vi "test15-LosslessRegisterStatusMultipleTimes.vi"(8 "error in (no error)":errorcluster, 11 "TestCase in":refnum<class "testcase-CSMBroadcast.lvclass">) -> (0 "error out":errorcluster, 3 "TestCase out":refnum<class "testcase-CSMBroadcast.lvclass">)   [LabVIEW 2017, in "testcase-CSMBroadcast.lvclass"]
uses:
  testcase-CSMBroadcast.lvclass
  bc269a46-fbd8-4fbd-ac76-06990d02385a.vi
  8d37a2f4-20d8-4102-818c-5a8acec6f80e.vi
  src/user.lib/_NEVSTOP/Communicable State Machine(CSM)/AdvanceAPI/CSM - Get Module Attribute.vi
  <vilib>/addons/_JKI Toolkits/VI Tester/TestCase.llb/TestCase.lvclass
  src/user.lib/_NEVSTOP/Communicable State Machine(CSM)/Communicable State Machine.lvlib
  CSM/CSM-Testcase.lvlib
  C:/Program Files (x86)/National Instruments/LabVIEW 2017/vi.lib/addons/_JKI Toolkits/VI Tester/TestCase.llb/TestCase.lvclass
panel:
  out "LoopCount":i32
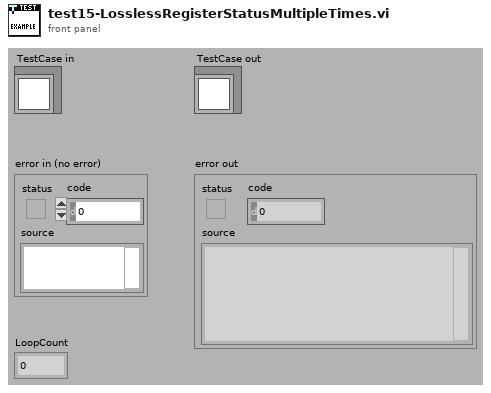
[diagram p1: front panel]
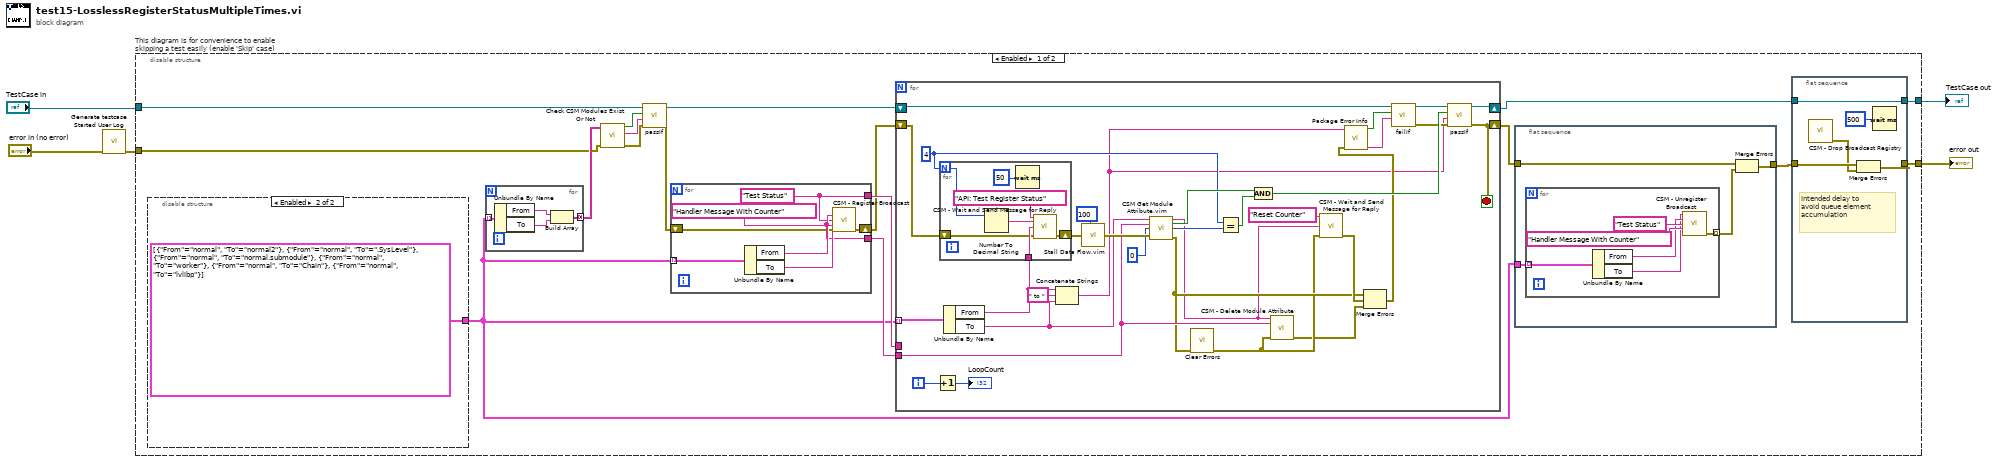
[diagram p0: block diagram]
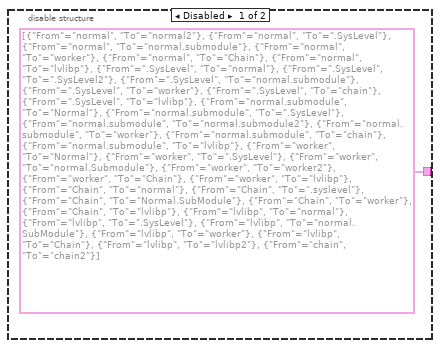
[diagram p2: hidden frame]
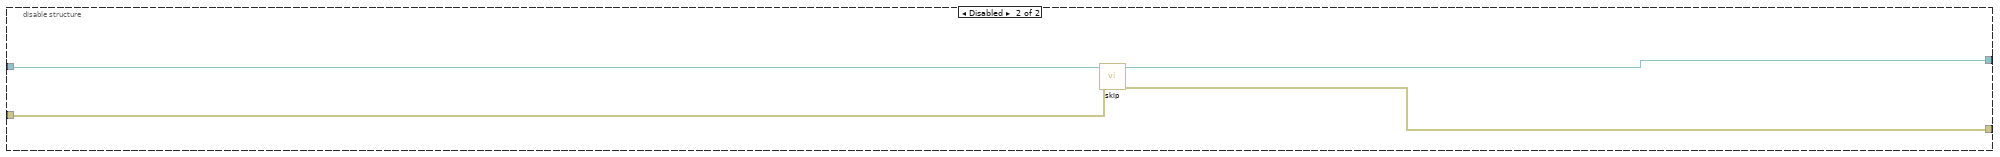
[diagram p3: hidden frame]
diagram:
  n1 = call "Generate testcase Started User Log.vi"("Error In"="error in (no error)") -> ("error out"=w1:errorcluster)  [unwired: 10 in]
  n2 = disable-structure "This diagram is for convenience to enable skipping a test easily (enable 'Skip' case)" shown="Enabled" {
    disable-tunnel: "TestCase in" -> [w11 w93]
    disable-tunnel: [w17 w91] -> w3
    disable-tunnel: [w20 w92] -> w2
    disable-tunnel: w1 -> [w9 w90]
    frame Enabled {
      n3 = disable-structure shown="Enabled" {
        disable-tunnel: [cluster{"From":string, "To":string}[] [{"From"="normal", "To"="normal2"}, {"From"="normal", "To"=".SysLevel"}, {"From"="normal", "To"="normal.submodule"}, {"From"="normal", "To"="worker"}, {"From"="normal", "To"="Chain"}, {"From"="normal", "To"="lvlibp"}, {"From"=".SysLevel", "To"="normal"}, {"From"=".SysLevel", "To"=".SysLevel2"}, {"From"=".SysLevel", "To"="normal.submodule"}, {"From"=".SysLevel", "To"="worker"}, {"From"=".SysLevel", "To"="chain"}, {"From"=".SysLevel", "To"="lvlibp"}, {"From"="normal.submodule", "To"="Normal"}, {"From"="normal.submodule", "To"=".SysLevel"}, {"From"="normal.submodule", "To"="normal.submodule2"}, {"From"="normal.submodule", "To"="worker"}, {"From"="normal.submodule", "To"="chain"}, {"From"="normal.submodule", "To"="lvlibp"}, {"From"="worker", "To"="Normal"}, {"From"="worker", "To"=".SysLevel"}, {"From"="worker", "To"="normal.Submodule"}, {"From"="worker", "To"="worker2"}, {"From"="worker", "To"="Chain"}, {"From"="worker", "To"="lvlibp"}, {"From"="Chain", "To"="normal"}, {"From"="Chain", "To"=".syslevel"}, {"From"="Chain", "To"="Normal.SubModule"}, {"From"="Chain", "To"="worker"}, {"From"="Chain", "To"="lvlibp"}, {"From"="lvlibp", "To"="normal"}, {"From"="lvlibp", "To"=".SysLevel"}, {"From"="lvlibp", "To"="normal.SubModule"}, {"From"="lvlibp", "To"="worker"}, {"From"="lvlibp", "To"="Chain"}, {"From"="lvlibp", "To"="lvlibp2"}, {"From"="chain", "To"="chain2"}] cluster{"From":string, "To":string}[] [{"From"="normal", "To"="normal2"}, {"From"="normal", "To"=".SysLevel"}, {"From"="normal", "To"="normal.submodule"}, {"From"="normal", "To"="worker"}, {"From"="normal", "To"="Chain"}, {"From"="normal", "To"="lvlibp"}]] -> w6
        frame Disabled {
        }
        frame Enabled {
        }
      }
      n4 = for {
        tunnel: w6 -> [w28] mode=indexing
        tunnel: [w25] -> w14 mode=concatenating
        n5 = Unbundle By Name(w28) -> ("From"=w27:string, "To"=w26:string)
        n6 = Build Array(w27, w26) -> (w25:string[])
      }
      n7 = call "Check CSM Modules Exist Or Not.vi"("error in"=w9, "CSM names in"=w14) -> ("error out"=w12:errorcluster, "Debug string"=w13:string, "All Modules Exist?"=w15:bool)  [unwired: 7 in]
      n8 = call-dynamic "passIf.vi"("error in (no error)"=w12, "message (\"\")"=w13, "pass"=w15, "TestCase in"=w11) -> ("error out"=w8:errorcluster, "TestCase out"=w10:refnum<class "testcase-CSMBroadcast.lvclass">)  [unwired: 6 in]
      n9 = for {
        tunnel: w6 -> [w45] mode=indexing
        tunnel: [w41] -> w19
        tunnel: [w40] -> w16
        shift-right: [w42] -> w7
        shift-left: w8 -> [w39]
        w40 = "Handler Message With Counter" ("Response Message (If \"\", Same as Source Message)")
        w41 = "Test Status" ("Status")
        n10 = Unbundle By Name(w45) -> ("From"=w44:string, "To"=w43:string)
        n11 = call "CSM - Register Broadcast.vi"("CSM Name(Empty for Broadcast Event)"=w43, "Source CSM Name (* as Default)"=w44, "Trigger"=w41, "API (If \"\", Same as Trigger)"=w40, "Error In"=w39) -> ("error out"=w42:errorcluster)  [unwired: 9 in, 1 out]
      }
      n12 = for {
        tunnel: w6 -> [w82] mode=indexing
        shift-right: [w77] -> w18
        shift-left: w10 -> [w60]
        shift-right: [w75] -> w22
        shift-left: w7 -> [w63]
        tunnel: w19 -> [_]
        tunnel: w16 -> [w74]
        i -> [w73]
        stop <- w75 stop-if-true
        w69 = 4
        n13 = Increment(x=w73) -> (x+1=→"LoopCount":i32)
        n14 = Unbundle By Name(w82) -> ("From"=w56:string, "To"=w55:string)
        n15 = for {
          N: w69 -> [w84]
          tunnel: w56 -> [w87]
          shift-right: [w88] -> w81
          shift-left: w63 -> [w86]
          n16 = Number To Decimal String(number=w84) -> (decimal integer string=w85:string)  [unwired: 1 in]
          n17 = Wait (ms)(milliseconds to wait=u32 50) -> ()  [unwired: 1 out]
          n18 = call "CSM - Wait and Send Message for Reply.vi"("State"="API: Test Register Status", "Arguments (\"\")"=w85, "Target Module"=w87, "Error In (No Error)"=w86) -> ("error out"=w88:errorcluster)  [unwired: 8 in, 3 out]
        }
        n19 = Concatenate Strings(w56, " to " ("string"), w55) -> (w53:string)
        n20 = call "Stall Data Flow.vim"("value in"=w81, "milliseconds to wait"=u32 100) -> ("value out"=w79:errorcluster)  [unwired: 1 out]
        n21 = call "CSM Get Module Attribute.vim"("CSM Name"=w55, "Attribute"=w74, "Default Value (Empty Variant)"=u32 0, "Error In"=w79) -> ("CSM Name (Dup)"=w51:string, "Found"=w78:bool, "Value"=w70:u32, "error out"=w66:errorcluster)  [unwired: 7 in, 1 out]
        n22 = call <vilib>:"Clear Errors.vi"("error in (no error)"=w66) -> ("error out"=w65:errorcluster)  [unwired: 5 in, 1 out]
        n23 = Equal?(x=w69, y=w70) -> (x = y?=w68:bool)
        n24 = Compound Arithmetic op=AND(w78, w68) -> (w76:bool)
        n25 = call "CSM - Delete Module Attribute.vi"("CSM Name"=w51, "Attribute"=w74, "Error In"=w65) -> ("error out"=w64:errorcluster)  [unwired: 9 in, 3 out]
        n26 = call "CSM - Wait and Send Message for Reply.vi"("State"="Reset Counter", "Target Module"=w51, "Error In (No Error)"=w65) -> ("error out"=w67:errorcluster)  [unwired: 9 in, 3 out]
        n27 = Merge Errors(w66, w67, w64) -> (w57:errorcluster)
        n28 = call "Package Error Info.vi"("error in"=w57, "String in"=w53) -> ("packed error info out"=w61:string, "error status"=w62:bool)  [unwired: 8 in]
        n29 = call-dynamic "failIf.vi"("message (\"\")"=w61, "fail"=w62, "TestCase in"=w60) -> ("error out"=w58:errorcluster, "TestCase out"=w59:refnum<class "testcase-CSMBroadcast.lvclass">)  [unwired: 7 in]
        n30 = call-dynamic "passIf.vi"("error in (no error)"=w58, "message (\"\")"=w53, "pass"=w76, "TestCase in"=w59) -> ("error out"=w75:errorcluster, "TestCase out"=w77:refnum<class "testcase-CSMBroadcast.lvclass">)  [unwired: 6 in]
      }
      n31 = flat-sequence {
        tunnel: w6 -> [w29]
        tunnel: w22 -> [w32]
        tunnel: [w31] -> w21
        frame #0 {
          n32 = for {
            tunnel: w29 -> [w33] mode=indexing
            tunnel: [w34] -> w30 mode=indexing
            n33 = Unbundle By Name(w33) -> ("From"=w36:string, "To"=w35:string)
            n34 = call "CSM - Unregister Broadcast.vi"("CSM Name(Empty for Broadcast Event)"=w35, "Source CSM Name (* as Default)"=w36, "Trigger"="Test Status" ("Status"), "API (\"*\" as Default)"="Handler Message With Counter" ("Response Message (If \"\", Same as Source Message)")) -> ("error out"=w34:errorcluster)  [unwired: 10 in, 1 out]
          }
          n35 = Merge Errors(w32, w30) -> (w31:errorcluster)
        }
      }
      n36 = flat-sequence {
        tunnel: w21 -> [w50]
        tunnel: [w49] -> w20
        tunnel: [w48] -> w17
        tunnel: w18 -> [w48]
        frame #0 {
          # "Intended delay to \navoid queue element\naccumulation"
          n37 = call "CSM - Drop Broadcast Registry.vi"() -> ("error out"=w47:errorcluster)  [unwired: 15 in]
          n38 = Merge Errors(w50, w47) -> (w49:errorcluster)
          n39 = Wait (ms)(milliseconds to wait=u32 500) -> ()  [unwired: 1 out]
        }
      }
    }
    frame Disabled {
      # "skip test result while test is under development"
      n40 = call <vilib>:"skip.vi"("error in (no error)"=w90, "TestCase in"=w93) -> ("error out"=w92:errorcluster, "TestCase out"=w91:refnum<class "testcase-CSMBroadcast.lvclass">)  [unwired: 8 in]
    }
  }
  "error out" <- w2
  "TestCase out" <- w3
